vi "full_stop_sequence.vi"(8 "error in":errorcluster, 11 "Queue in":refnum<queue>) -> (0 "error out":errorcluster, 3 "queue out":refnum<queue>)   [LabVIEW 2012]
uses:
  typedefs/MicroscopeEvent.ctl
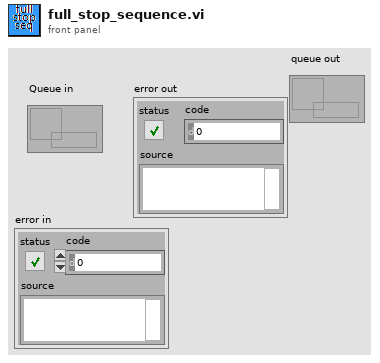
[diagram p1: front panel]
types:
  T1 = typedef "MicroscopeEvent.ctl" = enum16{"M.Wait", "M.RunRotation", "M.Flush", "M.Init", "M.InitStage", "M.InitImageData", "M.ReinitImageData", "M.ReinitImageParams", "M.GetSetParams", "M.InitFastHardware", "M.Pre-Acquire", "M.Acquire", "M.PostAcquire", "M.StopAcquire", "M.SetAcqStatusTrue", "M.SetAcqStatusFalse", "M.ClearImageData", "M.MoveStageDiscrete", "M.MoveStageToTarget1", "M.MoveStageToTarget2", "M.MoveStageToTarget3", "M.OpenShutters", "M.CloseShutters", "M.StartAcquireSequence", "M.ChangeParameters", "M.OpenStokes", "M.OpenPump", "M.RunSW"}
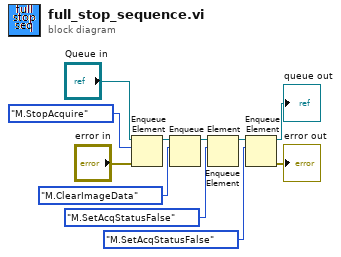
[diagram p0: block diagram]
diagram:
  n1 = Enqueue Element(queue="Queue in", element=MicroscopeEvent."M.StopAcquire", error in (no error)="error in") -> (queue out=w9:refnum<queue>)  [unwired: 1 in, 2 out]
  n2 = Enqueue Element(queue=w9, element=MicroscopeEvent."M.ClearImageData") -> (queue out=w8:refnum<queue>)  [unwired: 2 in, 2 out]
  n3 = Enqueue Element(queue=w8, element=MicroscopeEvent."M.SetAcqStatusFalse") -> (queue out=w6:refnum<queue>)  [unwired: 2 in, 2 out]
  n4 = Enqueue Element(queue=w6, element=MicroscopeEvent."M.SetAcqStatusFalse") -> (queue out=→"queue out":refnum<queue>, error out=→"error out":errorcluster)  [unwired: 2 in, 1 out]
